vi "NR_LDPC_Encode_opt.vi"(4 "error in (no error)":errorcluster caption="错误输入（无错误）", 6 "EN_LDPC":dbl, 7 "C":dbl=5.0, 8 "cdblkseg_data":dbl[][](array[numeric])=array5x8448[42240 elements], 9 "LDPC_base_graph":dbl=1.0, 11 "appended path":path=path "C:/Users/ES-SW/Desktop/5Gphysicallayerlinkprotocolimplementation/01 TeacherVersion/MatlabCode") -> (0 "error out":errorcluster caption="错误输出", 1 "coded_data":dbl[][](array[numeric]), 2 "null_pos":dbl[][](array[numeric]), 3 "H":dbl[][](array[numeric]))   [LabVIEW 2015]
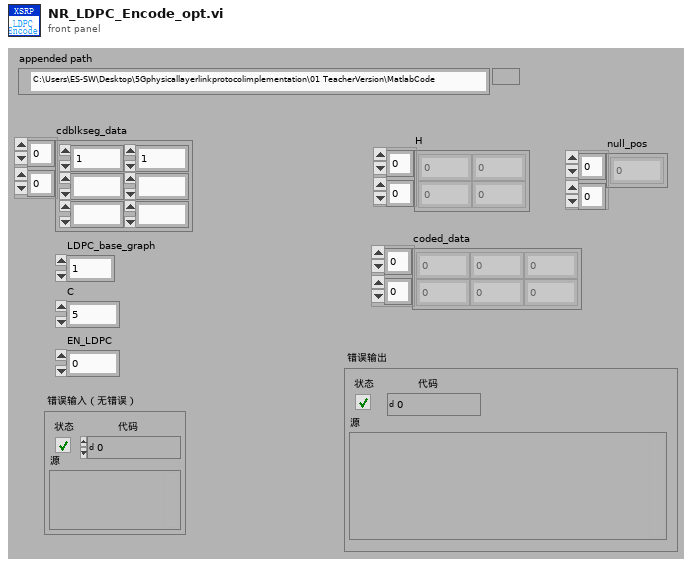
[diagram p1: front panel]
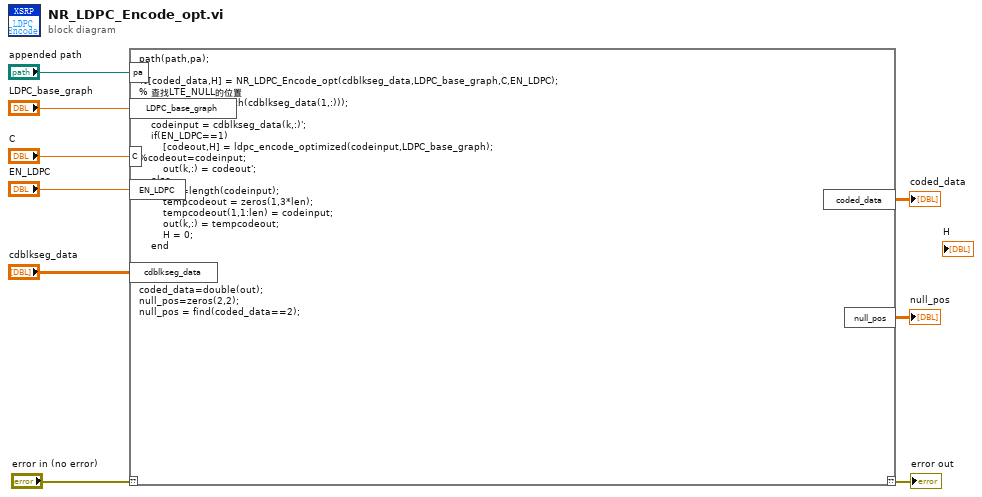
[diagram p0: block diagram]
diagram:
  n1 = script code="path(path,pa);\n\n%[coded_data,H] = NR_LDPC_Encode_opt(cdblkseg_data,LDPC_base_graph,C,EN_LDPC);\n% 查找LTE_NULL的位置\nout=zeros(C,3*length(cdblkseg_data(1,:)));\nfor k =1:C\n    codeinput = cdblkseg_data(k,:)';\n    if(EN_LDPC==1)\n        [codeout,H] = ldpc_encode_optimized(codeinput,LDPC_base_graph);\n%codeout=codeinput;\n        out(k,:) = codeout';\n    else\n        len =length(codeinput);\n        tempcodeout = zeros(1,3*len);\n        tempcodeout(1,1:len) = codeinput;\n        out(k,:) = tempcodeout;\n        H = 0;\n    end\n\nend\n\ncoded_data=double(out);\nnull_pos=zeros(2,2);\nnull_pos = find(coded_data==2);"("??"="error in (no error)", "pa"="appended path", "LDPC_base_graph"="LDPC_base_graph", "cdblkseg_data"="cdblkseg_data", "C"="C", "EN_LDPC"="EN_LDPC") -> ("??"=→"error out":errorcluster, "coded_data"=→"coded_data":dbl[][], "null_pos"=→"null_pos":dbl[][])
